vi "Get Auton Command VI.vi"(1 "Autonomous Command Name":T1) -> (0 "VI Refnum":refnum<vi>)   [LabVIEW 2014]
uses:
  Autonomous Commands/Autonomous Command Names.ctl
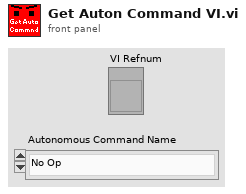
[diagram p1: front panel]
types:
  T1 = typedef "Autonomous Command Names.ctl" = enum16{"No Op", "Drive Distance Robot", "Drive Time Robot", "Translate Distance Robot", "Translate Time Robot", "Drive Distance Field", "Drive Time Field", "Translate Distance Field", "Translate Time Field", "Rotate Robot", "Set Initial Gyro Value", "Lifter to Setpoint", "Wait", "Do Not use", "Drive Distance Field (Gyro Hold)", "Translate Distance Field (Gyro Hold)", "Can", "Grabber", "Drive Distance Field (Sensor Stop, Gyro Hold)", "Move Direction Field (Gyro Hold)", "Rotate Robot 90 about Tote", "Reset Gyro", "Find Tote", "Get Tote Into Robot", "Lower Can Grabber"}
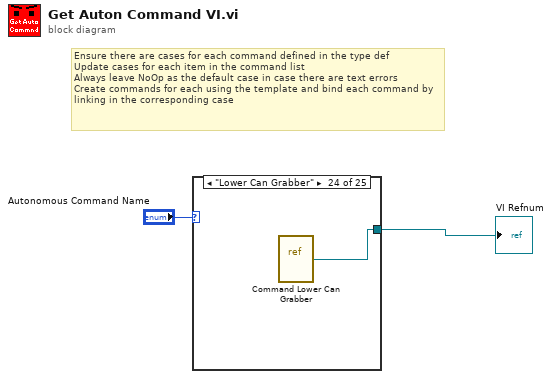
[diagram p0: block diagram]
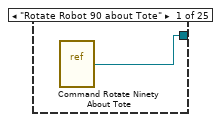
[diagram p2: hidden frame]
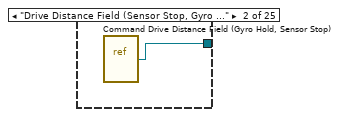
[diagram p3: hidden frame]
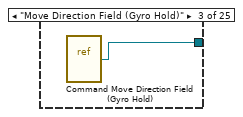
[diagram p4: hidden frame]
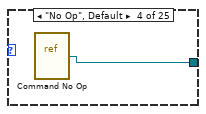
[diagram p5: hidden frame]
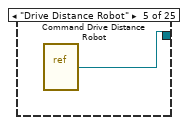
[diagram p6: hidden frame]
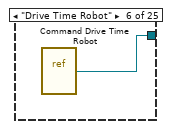
[diagram p7: hidden frame]
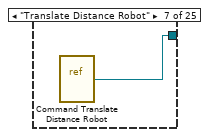
[diagram p8: hidden frame]
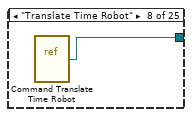
[diagram p9: hidden frame]
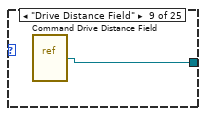
[diagram p10: hidden frame]
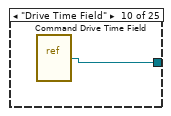
[diagram p11: hidden frame]
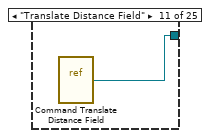
[diagram p12: hidden frame]
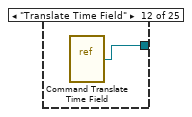
[diagram p13: hidden frame]
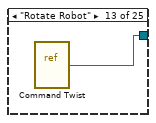
[diagram p14: hidden frame]
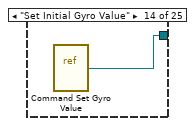
[diagram p15: hidden frame]
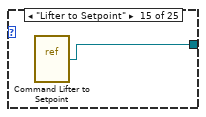
[diagram p16: hidden frame]
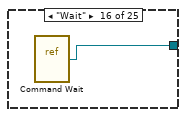
[diagram p17: hidden frame]
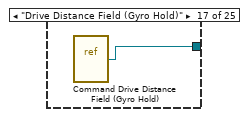
[diagram p18: hidden frame]
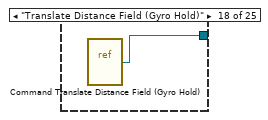
[diagram p19: hidden frame]
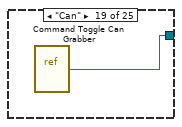
[diagram p20: hidden frame]
diagram:
  # "Ensure there are cases for each command defined in the type def\nUpdate cases for each item in the command list\nAlways leave NoOp as the default case in case there are text errors\nCreate commands for each using the template and bind each command by linking in the corresponding case"
  n1 = case shown="\"Lower Can Grabber\"" "Autonomous Command Name" {
    tunnel: [w3 w4 w5 w6 w7 w8 w9 w10 w11 w12 w13 w14 w15 w16 w17 w18 w19 w20 w21 w22 w23 w24 w25 w26 w27] -> w1
    frame "Rotate Robot 90 about Tote" {
      n2 = vi-ref "Command Rotate Ninety About Tote.vi"() -> (w3:refnum<vi>)
    }
    frame "Drive Distance Field (Sensor Stop, Gyro Hold)" {
      n3 = vi-ref "Command Drive Distance Field (Gyro Hold, Sensor Stop).vi"() -> (w4:refnum<vi>)
    }
    frame "Move Direction Field (Gyro Hold)" {
      n4 = vi-ref "Command Move Direction Field (Gyro Hold).vi"() -> (w5:refnum<vi>)
    }
    frame "No Op", Default {
      n5 = vi-ref "Command No Op.vi"() -> (w6:refnum<vi>)
    }
    frame "Drive Distance Robot" {
      n6 = vi-ref "Command Drive Distance Robot.vi"() -> (w7:refnum<vi>)
    }
    frame "Drive Time Robot" {
      n7 = vi-ref "Command Drive Time Robot.vi"() -> (w8:refnum<vi>)
    }
    frame "Translate Distance Robot" {
      n8 = vi-ref "Command Translate Distance Robot.vi"() -> (w9:refnum<vi>)
    }
    frame "Translate Time Robot" {
      n9 = vi-ref "Command Translate Time Robot.vi"() -> (w10:refnum<vi>)
    }
    frame "Drive Distance Field" {
      n10 = vi-ref "Command Drive Distance Field.vi"() -> (w11:refnum<vi>)
    }
    frame "Drive Time Field" {
      n11 = vi-ref "Command Drive Time Field.vi"() -> (w12:refnum<vi>)
    }
    frame "Translate Distance Field" {
      n12 = vi-ref "Command Translate Distance Field.vi"() -> (w13:refnum<vi>)
    }
    frame "Translate Time Field" {
      n13 = vi-ref "Command Translate Time Field.vi"() -> (w14:refnum<vi>)
    }
    frame "Rotate Robot" {
      n14 = vi-ref "Command Twist.vi"() -> (w15:refnum<vi>)
    }
    frame "Set Initial Gyro Value" {
      n15 = vi-ref "Command Set Gyro Value.vi"() -> (w16:refnum<vi>)
    }
    frame "Lifter to Setpoint" {
      n16 = vi-ref "Command Lifter to Setpoint.vi"() -> (w17:refnum<vi>)
    }
    frame "Wait" {
      n17 = vi-ref "Command Wait.vi"() -> (w18:refnum<vi>)
    }
    frame "Drive Distance Field (Gyro Hold)" {
      n18 = vi-ref "Command Drive Distance Field (Gyro Hold).vi"() -> (w19:refnum<vi>)
    }
    frame "Translate Distance Field (Gyro Hold)" {
      n19 = vi-ref "Command Translate Distance Field (Gyro Hold).vi"() -> (w20:refnum<vi>)
    }
    frame "Can" {
      n20 = vi-ref "Command Toggle Can Grabber.vi"() -> (w21:refnum<vi>)
    }
    frame "Grabber" {
      n21 = vi-ref "Command Toggle Lifter Fingers.vi"() -> (w22:refnum<vi>)
    }
    frame "Reset Gyro" {
      n22 = vi-ref "Command Reset Gyro.vi"() -> (w23:refnum<vi>)
    }
    frame "Find Tote" {
      n23 = vi-ref "Command Find Tote.vi"() -> (w24:refnum<vi>)
    }
    frame "Get Tote Into Robot" {
      n24 = vi-ref "Command Get Tote Into Robot.vi"() -> (w25:refnum<vi>)
    }
    frame "Lower Can Grabber" {
      n25 = vi-ref "Command Lower Can Grabber.vi"() -> (w26:refnum<vi>)
    }
    frame "Do Not use" {
      n26 = vi-ref "Command Get Tote Into Robot.vi"() -> (w27:refnum<vi>)
    }
  }
  "VI Refnum" <- w1
